vi "Read ENV for GET.vi"(2 "ENV":T1) -> (0 "GET query params":T1)   [LabVIEW 2011]
doc: "Returns the parameters that a CGI request contains. If the request contains a single parameter, the calling VI must use <B>query string</B>. If the request contains a list of parameters, the calling VI must use <B>query params</B>."
uses:
  ITK EXT/utils/keyedarr.llb/Keyed Array.ctl
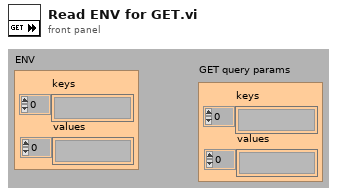
[diagram p1: front panel]
types:
  T1 = typedef "Keyed Array.ctl" = cluster{"keys":string[], "values":string[]}
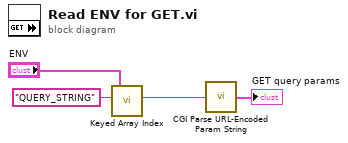
[diagram p0: block diagram]
diagram:
  n1 = call "Keyed Array Index.vi"("key"="QUERY_STRING" ("name"), "array in"="ENV") -> ("value"=w2:string)  [unwired: 2 in, 3 out]
  n2 = call "CGI Parse URL-Encoded Param String.vi"("url-encoded param string"=w2) -> ("params"=→"GET query params":T1)
